vi "API - Close Connection.vi"(8 "error in":errorcluster, 11 "DAQiFi Device Properties In":T1) -> (0 "error out":errorcluster, 3 "DAQiFi Device Properties Out":T1)   [LabVIEW 2021]
doc: "Stop any data streaming and close the connection to the DAQ."
uses:
  TypeDefs/TypeDef - Cluster of DAQiFi Device Properties.ctl
  TypeDefs/Enum - Connection Type.ctl
  TCP - Asynchronous Write.vi
  USB - Asynchronous Write.vi
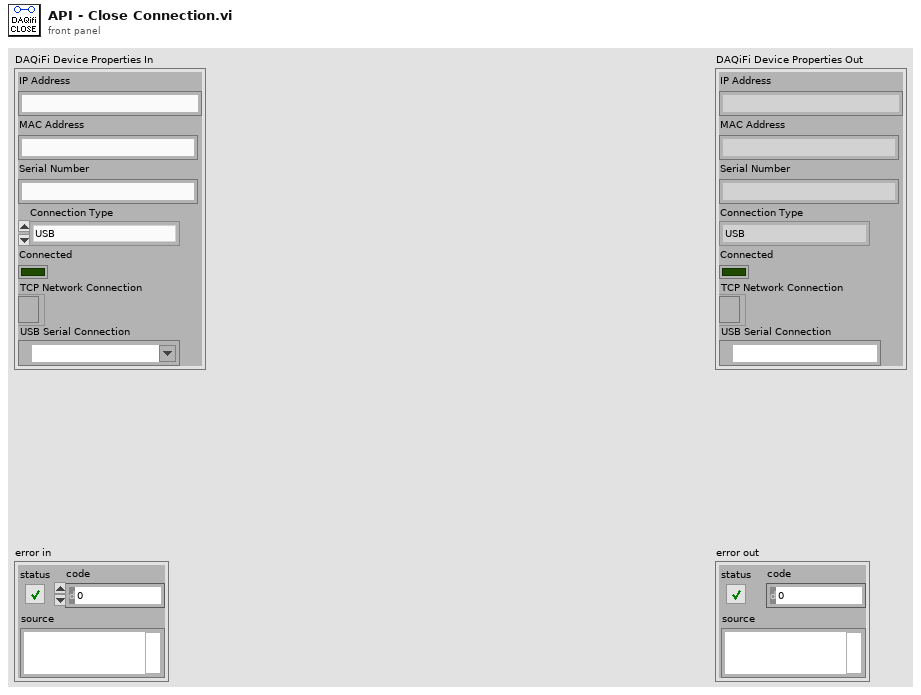
[diagram p1: front panel]
types:
  T1 = typedef "TypeDef - Cluster of DAQiFi Device Properties.ctl" = cluster{"IP Address":string, "MAC Address":string, "Serial Number":string, "Connection Type":T2, "Connected":bool, "TCP Network Connection":refnum<k5>, "USB Serial Connection":refnum<visa-resource-name>}
  T2 = typedef "Enum - Connection Type.ctl" = enum16{"USB", "TCP"}
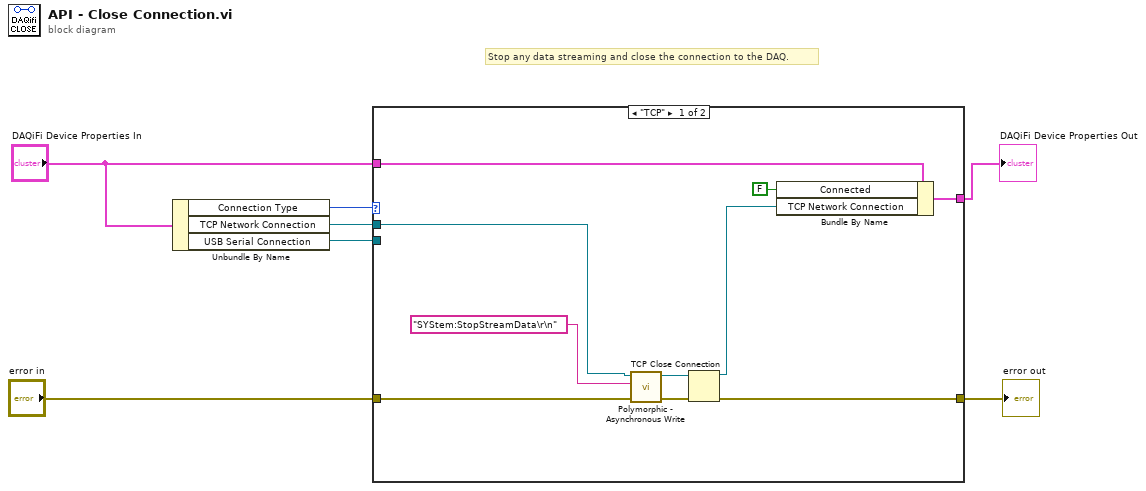
[diagram p0: block diagram]
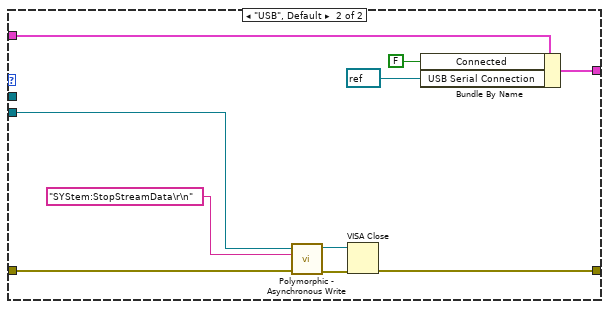
[diagram p2: hidden frame]
diagram:
  # "Stop any data streaming and close the connection to the DAQ."
  n1 = Unbundle By Name("DAQiFi Device Properties In") -> ("Connection Type"=w7:T2, "TCP Network Connection"=w6:refnum<k5>, "USB Serial Connection"=w1:refnum<visa-resource-name>)
  n2 = case shown="\"TCP\"" w7 {
    tunnel: w6 -> [w10 _]
    tunnel: "error in" -> [w12 w19]
    tunnel: [w17 w24] -> w4
    tunnel: "DAQiFi Device Properties In" -> [w16 w27]
    tunnel: [w13 w25] -> w2
    tunnel: w1 -> [_ w22]
    frame "TCP" {
      n3 = call-poly "Polymorphic - Asynchronous Write.vi"("error in"=w12, "Message to Send"="SYStem:StopStreamData\r\n", "TCP Network Connection in"=w10) -> ("error out"=w8:errorcluster, "TCP Network Connection out"=w9:refnum<k5>)  [unwired: 7 in]
      n4 = TCP Close Connection(connection ID=w9, error in (no error)=w8) -> (connection ID out=w14:refnum<k5>, error out=w17:errorcluster)  [unwired: 1 in]
      n5 = Bundle By Name(cluster=w16, "Connected"=FALSE, "TCP Network Connection"=w14) -> (w13:T1)
    }
    frame "USB", Default {
      n6 = call-poly "Polymorphic - Asynchronous Write.vi"("error in"=w19, "Message to Send"="SYStem:StopStreamData\r\n", "VISA resource name in"=w22) -> ("error out"=w18:errorcluster, "VISA resource name out"=w21:refnum<visa-resource-name>)  [unwired: 7 in]
      n7 = VISA Close(VISA resource name=w21, error in (no error)=w18) -> (error out=w24:errorcluster)
      n8 = Bundle By Name(cluster=w27, "Connected"=FALSE, "USB Serial Connection"=refnum<visa-resource-name> refnum) -> (w25:T1)
    }
  }
  "error out" <- w4
  "DAQiFi Device Properties Out" <- w2
